vi "RT Host - calc step x & y.vi"(6 "Max Step Inc (mm)":dbl, 8 "error in (no error)":errorcluster, 10 "Previous Target Global W/S Pos (mm)":dbl[](array[numeric])=[0.0, -90.0], 11 "Target Global W/S Pos (mm)":dbl[](array[numeric])=[0.0, -90.0]) -> (0 "error out":errorcluster, 1 "Max Y Increment (mm)":dbl, 2 "Max X Increment (mm)":dbl)   [LabVIEW 2017]
doc: "This subVI is used to work out the max X and Y step increment per iteration."
panel:
  # "Outputs"
  # "Inputs"
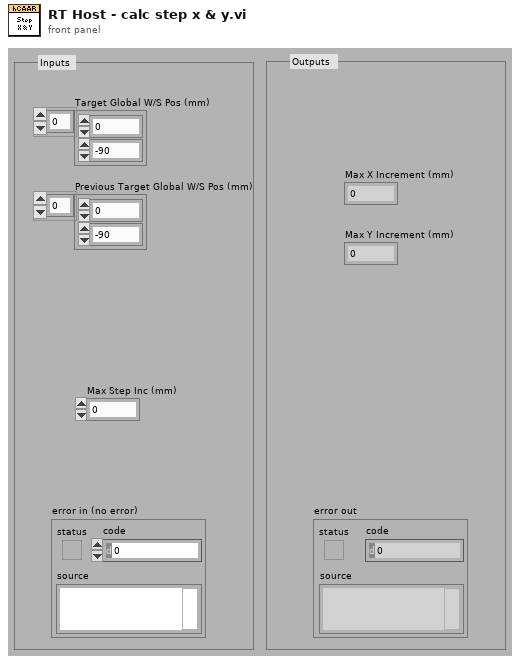
[diagram p1: front panel]
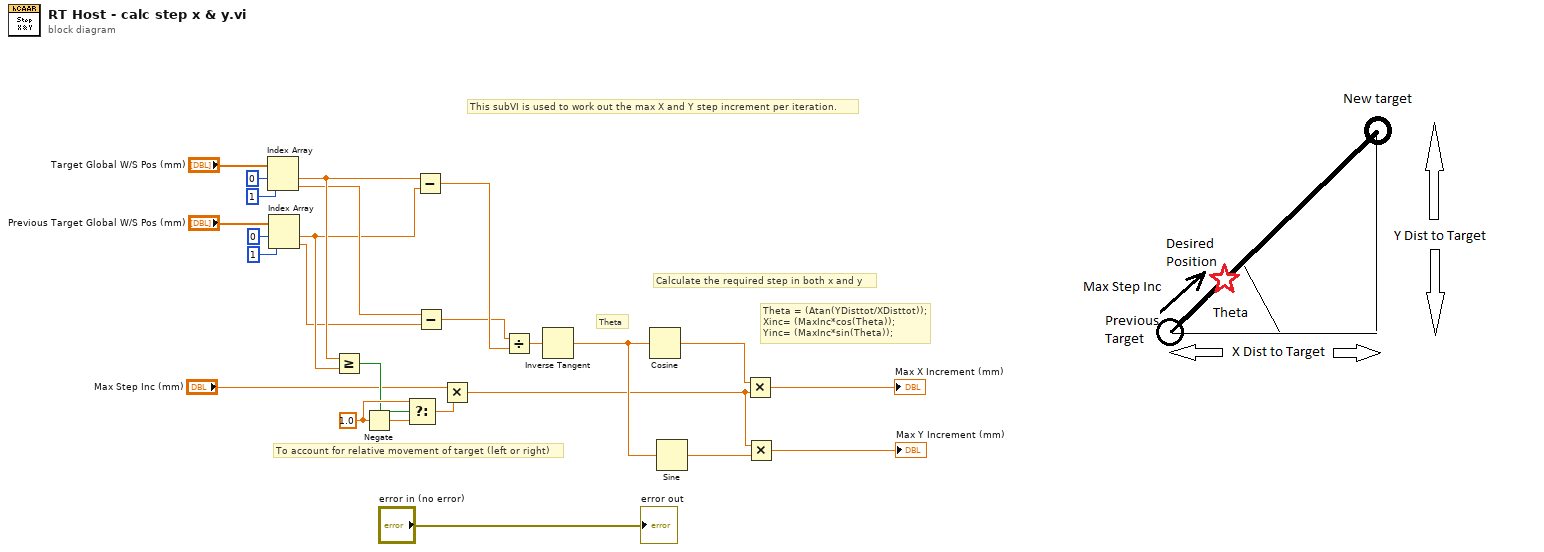
[diagram p0: block diagram]
diagram:
  w15 = 1.0 ("f")
  # "To account for relative movement of target (left or right)"
  # "Theta"
  # "Theta = (Atan(YDisttot/XDisttot));\nXinc= (MaxInc*cos(Theta));\nYinc= (MaxInc*sin(Theta));"
  # "Calculate the required step in both x and y"
  # "This subVI is used to work out the max X and Y step increment per iteration."
  n1 = Index Array(array="Target Global W/S Pos (mm)", index #1=0 ("index"), index #2=1 ("index")) -> (element #1=w5:dbl, element #2=w4:dbl)
  n2 = Index Array(array="Previous Target Global W/S Pos (mm)", index #1=0 ("index"), index #2=1 ("index")) -> (element #1=w3:dbl, element #2=w2:dbl)
  n3 = Greater Or Equal?(x=w5, y=w3) -> (x >= y?=w14:bool)
  n4 = Negate(x=w15) -> (-x=w16:dbl)
  n5 = Select(t=w15, s=w14, f=w16) -> (s? t:f=w17:dbl)
  n6 = Subtract(x=w5, y=w3) -> (x-y=w19:dbl)
  n7 = Subtract(x=w4, y=w2) -> (x-y=w18:dbl)
  n8 = Multiply(x="Max Step Inc (mm)", y=w17) -> (x*y=w12:dbl)
  n9 = Divide(x=w18, y=w19) -> (x/y=w20:dbl)
  n10 = Inverse Tangent(1:w20) -> (0:w22:dbl)
  n11 = Cosine(x=w22) -> (cos(x)=w21:dbl)
  n12 = Sine(x=w22) -> (sin(x)=w23:dbl)
  n13 = Multiply(x=w21, y=w12) -> (x*y=→"Max X Increment (mm)":dbl)
  n14 = Multiply(x=w12, y=w23) -> (x*y=→"Max Y Increment (mm)":dbl)
  "error out" <- "error in (no error)"
